vi "Main.vi"() -> ()   [LabVIEW 2017]
doc: "The program is for the real-time control of digital output pins on the Arduino Uno microcontroller.\n\nThe program is configured for the use of 6 DIO pins numbered 2-7. The pins can be be used to output AC and DC signals. The pins can also be swtiched on for a preset length of time."
uses:
  controls/UI Data.ctl
  <vilib>/MakerHub/LINX/Public/Peripherals/Digital/Digital Write 1 Chan.vi
  <vilib>/MakerHub/LINX/Public/Peripherals/Digital/Digital Write N Chans.vi
  <vilib>/MakerHub/LINX/Private/Local IO/LinxDigitalWrite.vi
  <vilib>/MakerHub/LINX/Public/Utilities/Check Channel.vi
  support/Message Queue/Enqueue Message (Single).vi
  <vilib>/MakerHub/LINX/Public/Utilities/Open Serial.vi
  <vilib>/MakerHub/LINX/Private/Utilties/Generate Error.vi
  <vilib>/Utility/error.llb/Error Cluster From Error Code.vi
  <vilib>/ErrorRing/Error Ring.xnode
  support/Message Queue/Message Queue.lvlib
  support/User Event - Stop/User Event - Stop.lvlib
  <vilib>/MakerHub/LINX/LMH-LINX.lvlib
panel:
  in  "Frequency (Hz)":dbl
  in  "DC/AC":bool
  in  "On-time (ms)":dbl
  in  "Start Button":bool
  in  "COM Port":refnum<visa-resource-name>="COM3"
  out "User Prompts":string="Initializing...."
  in  "Restart Button":bool
  in  "Exit":bool
  in  "Electrode Control":bool[][](array[boolean])=[[FALSE, FALSE, FALSE], [FALSE, FALSE, FALSE]]
  out "Error Out":errorcluster
  # "Digital Microfluidics HV Switching Control"
  # "Program Status"
  # "Timing Controls"
  # "DC"
  # "AC"
  # "Electrode Controls"
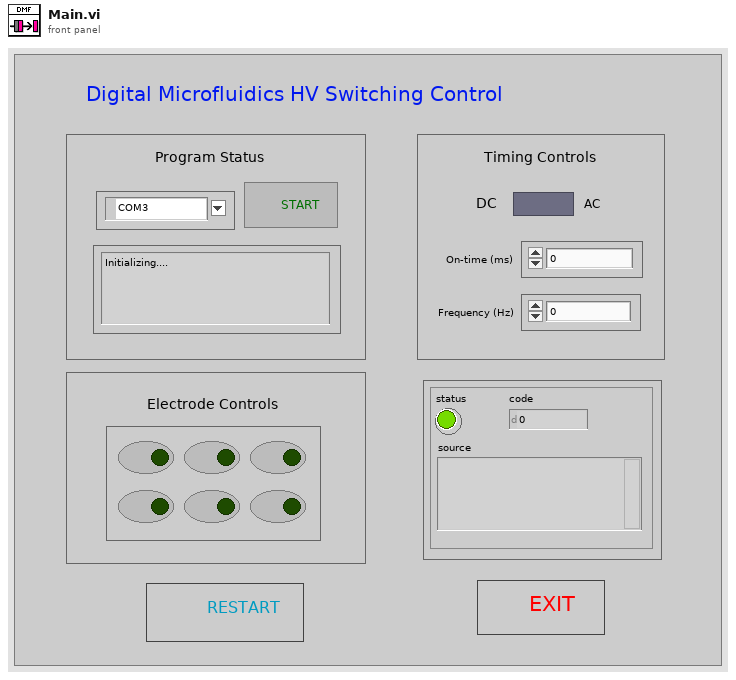
[diagram p1: front panel]
types:
  T1 = typedef "UI Data.ctl" = cluster{"VISA resource name":refnum<vi>, "Start Button":refnum<vi>, "DC/AC":refnum<vi>, "On-time (ms)":refnum<vi>, "Frequency (Hz)":refnum<vi>, "User Prompts":refnum<vi>, "Electrode Control":refnum<vi>, "Restart Button":refnum<vi>, "Exit":refnum<vi>}
  T2 = typedef "Message Queue.lvlib/All Message Queues.ctl" = cluster{"UI":refnum<queue>}
  T3 = typedef "LMH-LINX.lvlib/LINX Ref.ctl" = cluster{"IO":T4, "Interface":T5, "LINX Device Config":T6}
  T4 = typedef "LMH-LINX.lvlib/Platform.ctl" = enum16{"Remote", "Local"}
  T5 = typedef "LMH-LINX.lvlib/Interface.ctl" = enum16{"Serial", "TCP"}
  T6 = typedef "LMH-LINX.lvlib/Device.lvlib/LINX Device Config.ctl" = cluster{"Interface":T5, "COM Port":refnum<visa-resource-name>, "TCP Configuration":T7, "Device Family":u8, "Device ID":u8, "Device Name":string, "TCP Ref":refnum<k5>, "Channels":T8}
  T7 = typedef "LMH-LINX.lvlib/Device.lvlib/TCP Config.ctl" = cluster{"IP Address":string, "Port":u16}
  T8 = typedef "LMH-LINX.lvlib/Channels.ctl" = cluster{"DI":u8[], "DO":u8[], "AI":u8[], "AO":u8[], "PWM":u8[], "QE":u8[], "UART":u8[], "I2C 2":u8[], "SPI":u8[], "CAN":u8[], "Servo":u8[], "AI Ref (V)":dbl, "AI Resolution (Bits)":u8, "AO Ref (V)":dbl, "AO Resolution (Bits)":u8}
  T9 = cluster{i32, "index of element":i32, "Boolean":bool}
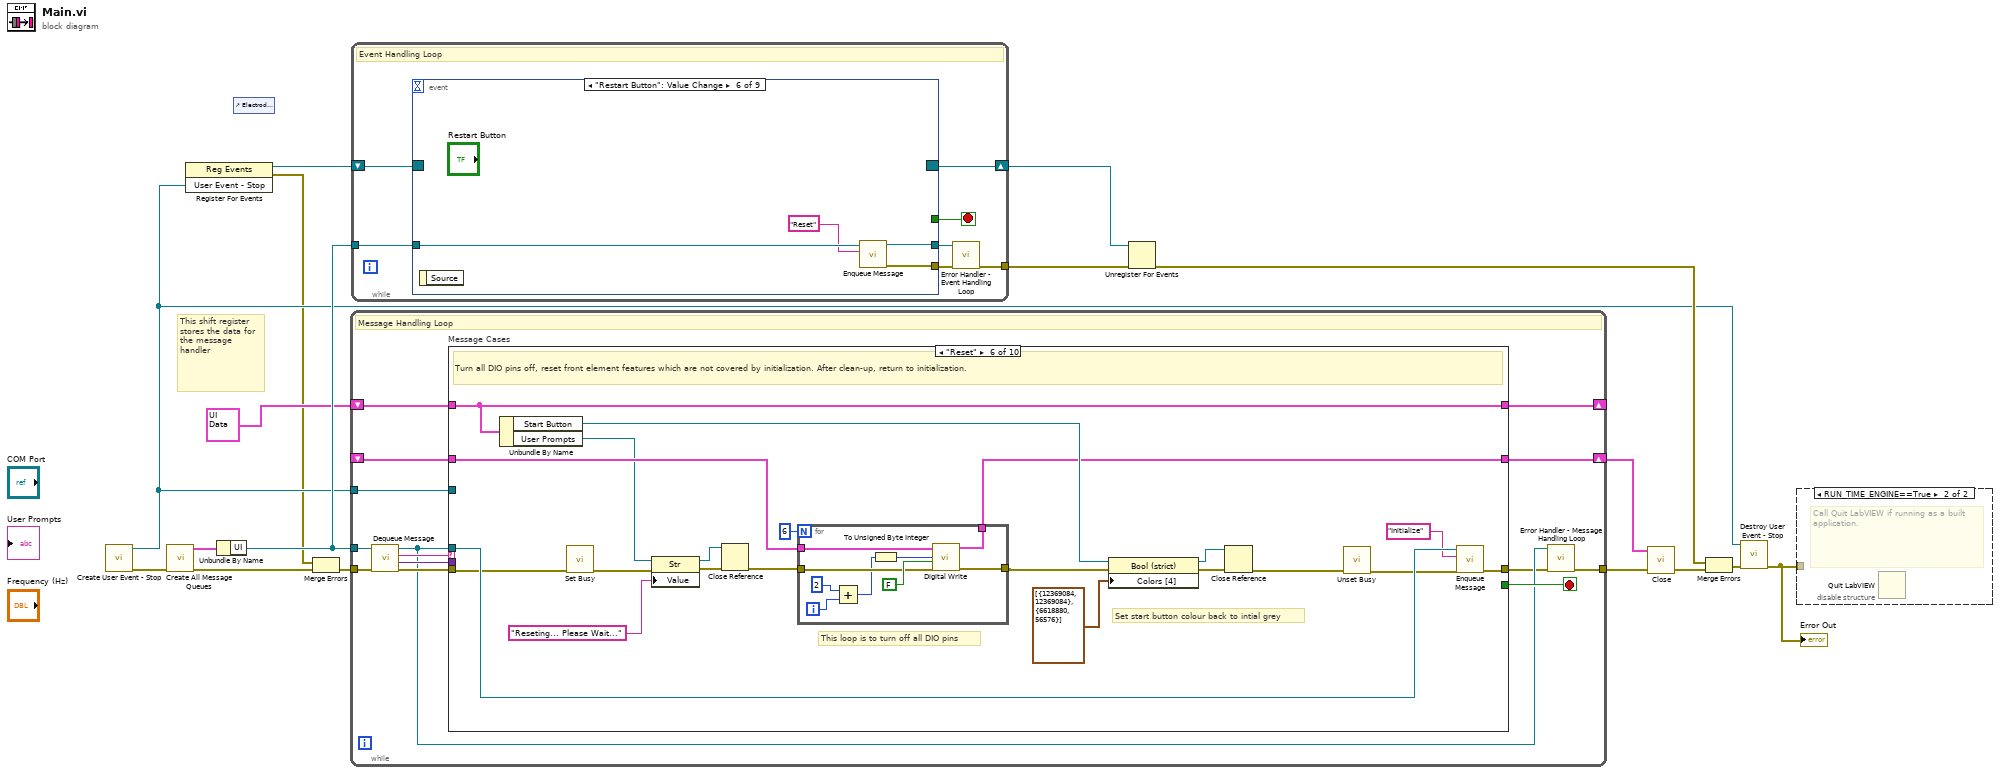
[diagram p0: block diagram]
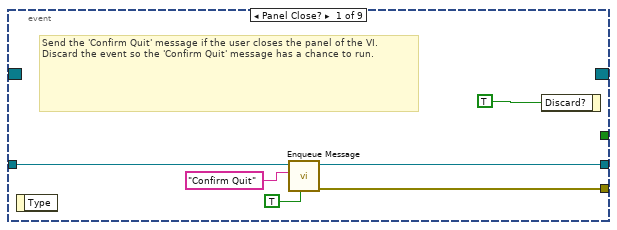
[diagram p3: hidden frame]
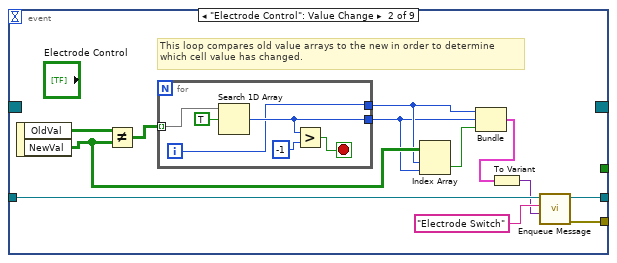
[diagram p4: hidden frame]
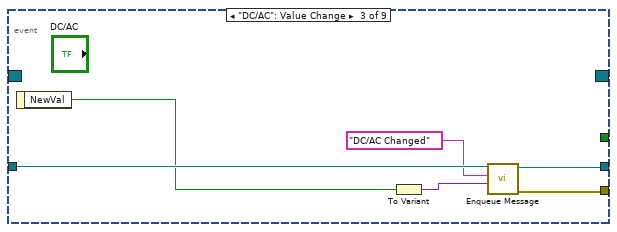
[diagram p5: hidden frame]
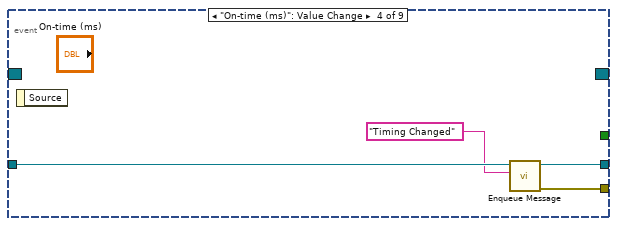
[diagram p6: hidden frame]
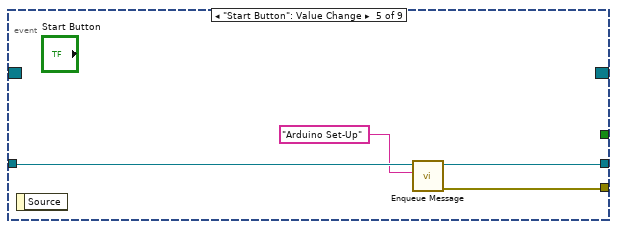
[diagram p7: hidden frame]
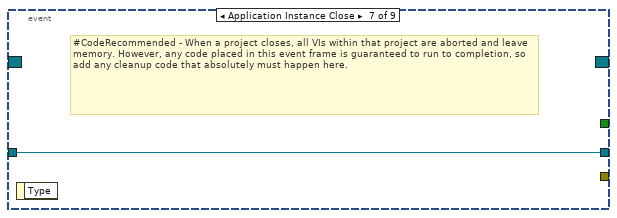
[diagram p8: hidden frame]
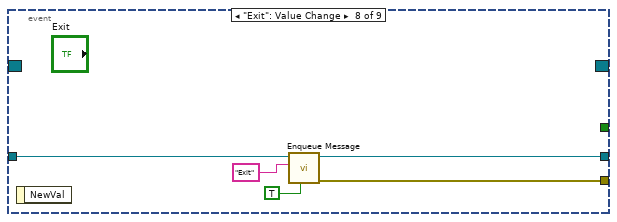
[diagram p9: hidden frame]
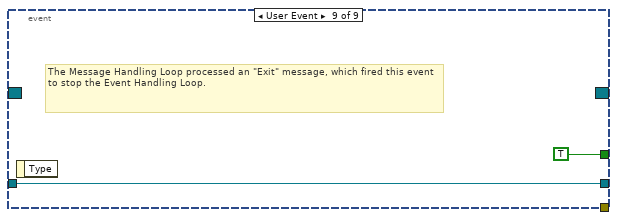
[diagram p10: hidden frame]
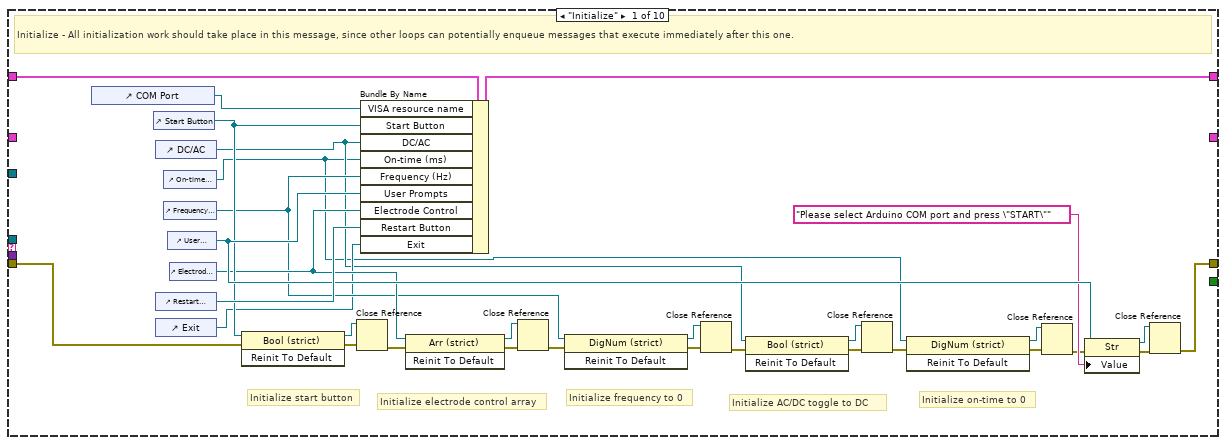
[diagram p11: hidden frame]
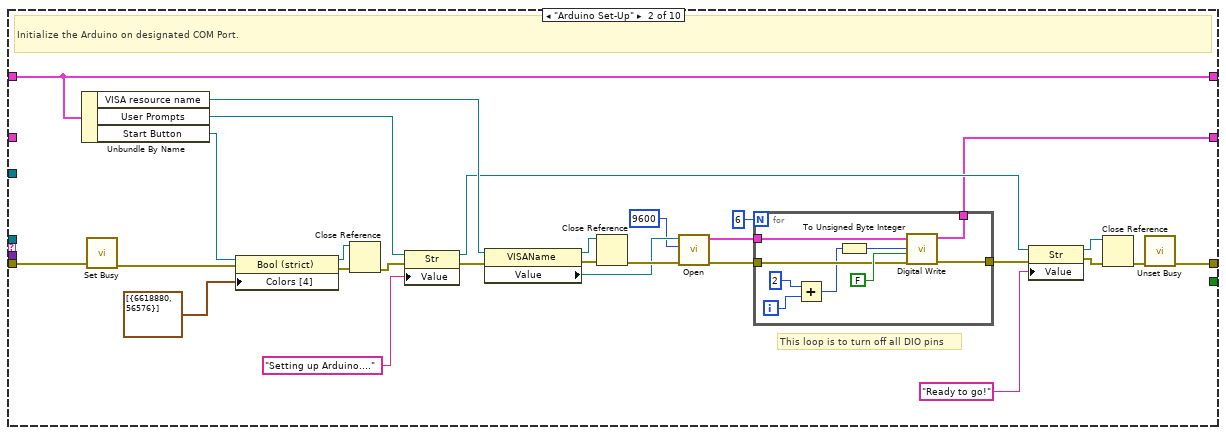
[diagram p12: hidden frame]
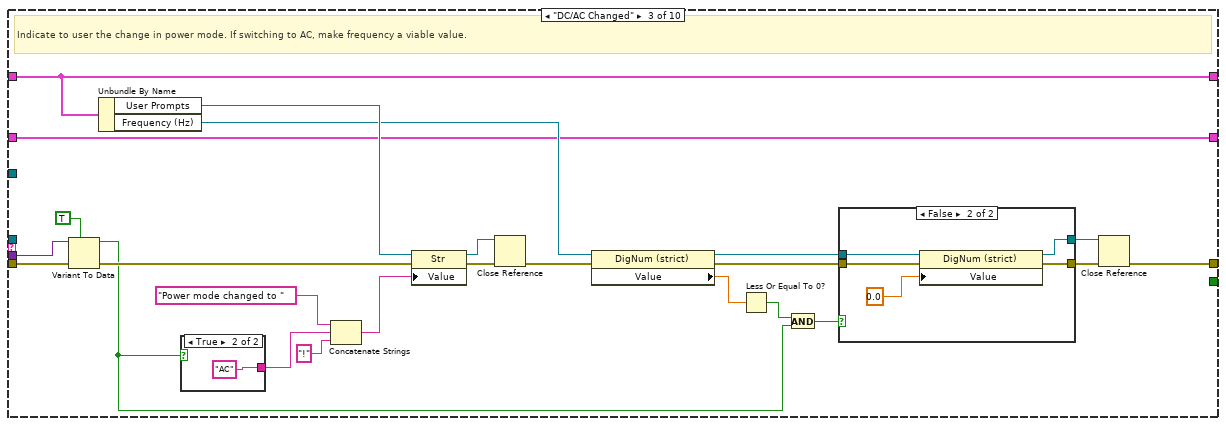
[diagram p13: hidden frame]
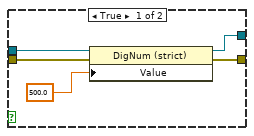
[diagram p14: hidden frame]
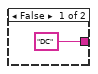
[diagram p15: hidden frame]
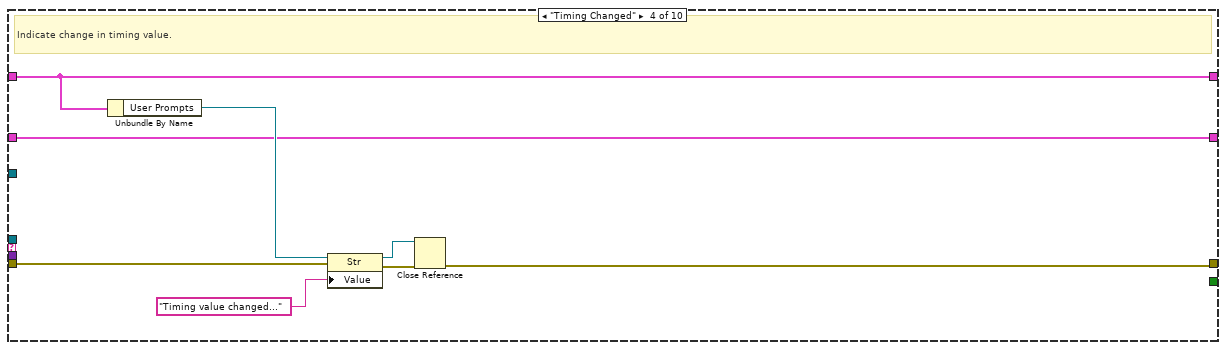
[diagram p16: hidden frame]
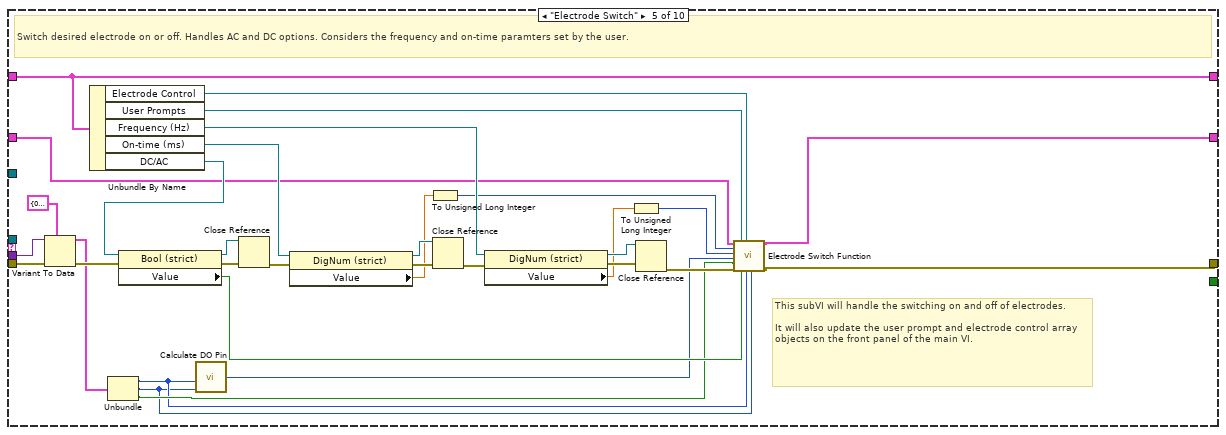
[diagram p17: hidden frame]
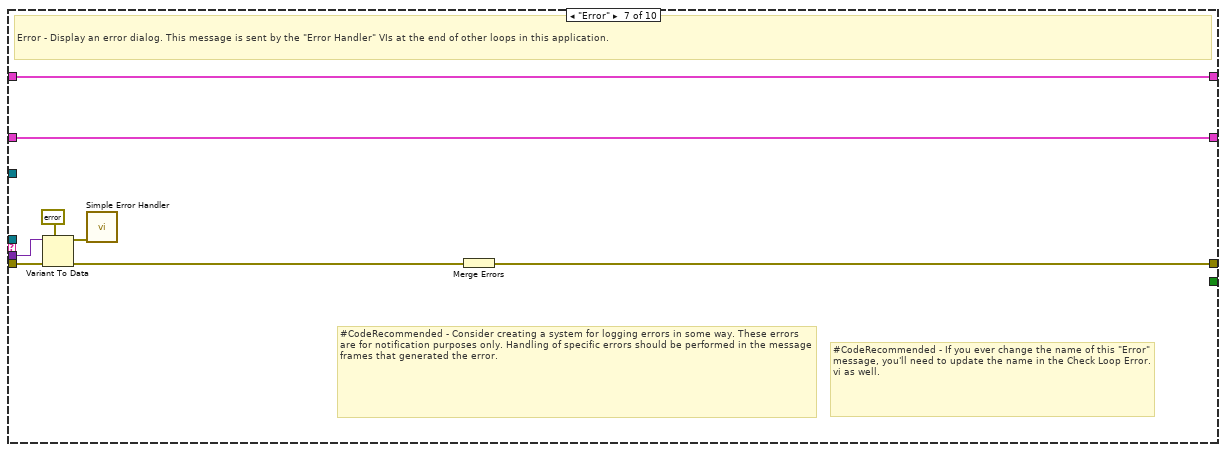
[diagram p18: hidden frame]
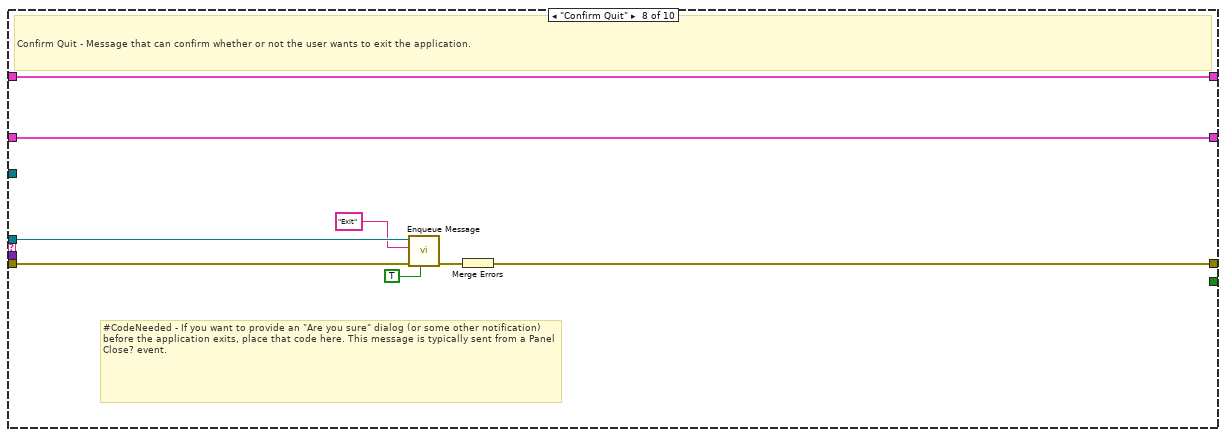
[diagram p19: hidden frame]
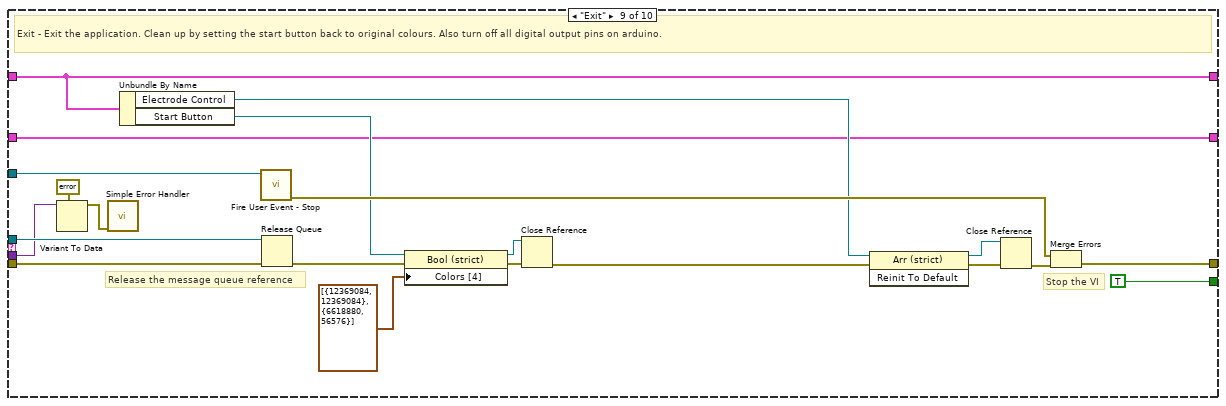
[diagram p20: hidden frame]
diagram:
  # "This shift register stores the data for the message handler"
  n1 = call "Create User Event - Stop.vi"() -> ("error out"=w14:errorcluster, "User Event - Stop"=w7:refnum<user-event>)  [unwired: 10 in]
  n2 = call "Create All Message Queues.vi"("error in (no error)"=w14) -> ("error out"=w17:errorcluster, "Message Queues out"=w16:T2)  [unwired: 9 in]
  n3 = register-events(w7) -> (reference out=w8:refnum<event-registration>, error out=w5:errorcluster)  [unwired: 2 in]
  n4 = Unbundle By Name(w16) -> ("UI"=w15:refnum<queue>)
  n5 = control-ref of="Electrode Control"() -> ()  [unwired: 1 out]
  n6 = Merge Errors(w5, w17) -> (w6:errorcluster)
  n7 = while {
    tunnel: w15 -> [w23]
    shift-right: [w30] -> _
    shift-left: T1 {"VISA resource name"=refnum, "Start Button"=refnum, "DC/AC"=refnum, "On-time (ms)"=refnum, "Frequency (Hz)"=refnum, "User Prompts"=refnum, "Electrode Control"=refnum, "Restart Button"=refnum, "Exit"=refnum} ("Data Cluster") -> [w31]
    tunnel: w7 -> [w28]
    tunnel: w6 -> [w27]
    tunnel: [w21] -> w3
    shift-right: [w19] -> w1
    shift-left: _ -> [w18]
    stop <- w29 stop-if-true
    # "Message Handling Loop"
    n8 = call "Dequeue Message.vi"("error in (no error)"=w27, "Message Queue"=w23) -> ("error out"=w26:errorcluster, "Message Data"=w24:variant, "Message"=w25:string, "dup Message Queue"=w22:refnum<queue>)  [unwired: 6 in]
    n9 = case "Message Cases" shown="\"Reset\"" w25 {
      selector: w25 -> [_ _ _ _ _ _ _ _ _ w244]
      tunnel: w22 -> [_ _ _ _ _ w187 _ w217 w242 _]
      tunnel: w26 -> [w53 w81 w122 w142 w175 w180 w213 w221 w237 _]
      tunnel: [w54 w79 w102 w138 w157 w188 w207 w219 w240 w245] -> w20
      tunnel: w31 -> [w62 w90 w123 w143 w172 w196 w212 w220 w233 w246]
      tunnel: [w61 w90 w123 w143 w172 w196 w212 w220 w233 w246] -> w30
      tunnel: [_ _ _ _ _ _ _ _ TRUE _] -> w29
      tunnel: w24 -> [_ _ w121 _ w174 _ w211 _ w234 _]
      tunnel: w28 -> [_ _ _ _ _ _ _ _ w239 _]
      tunnel: [_ w63 w100 w136 w156 w176 w206 w214 w223 w243] -> w19
      tunnel: w18 -> [_ _ w100 w136 w150 w194 w206 w214 w223 w243]
      frame "Initialize" {
        # "Initialize on-time to 0"
        # "Initialize AC/DC toggle to DC"
        # "Initialize frequency to 0"
        # "Initialize electrode control array"
        # "Initialize start button"
        # "Initialize - All initialization work should take place in this message, since other loops can potentially enqueue messages that execute immediately after this one."
        n10 = control-ref of="COM Port"() -> (w60:refnum<vi>)
        n11 = control-ref of="Start Button"() -> (w52:refnum<vi>)
        n12 = control-ref of="DC/AC"() -> (w39:refnum<vi>)
        n13 = control-ref of="Restart Button"() -> (w59:refnum<vi>)
        n14 = control-ref of="Exit"() -> (w41:refnum<vi>)
        n15 = control-ref of="On-time (ms)"() -> (w35:refnum<vi>)
        n16 = control-ref of="Frequency (Hz)"() -> (w44:refnum<vi>)
        n17 = control-ref of="User Prompts"() -> (w58:refnum<vi>)
        n18 = control-ref of="Electrode Control"() -> (w49:refnum<vi>)
        n19 = invoke class="Bool (strict)" method="Reinit To Default"(reference=w52, error in=w53) -> (reference out=w50:refnum<vi>, error out=w51:errorcluster)  [unwired: 1 in, 1 out]
        n20 = Close Reference(reference=w50, error in (no error)=w51) -> (error out=w48:errorcluster)
        n21 = Bundle By Name(cluster=w62, "VISA resource name"=w60, "Start Button"=w52, "DC/AC"=w39, "On-time (ms)"=w35, "Frequency (Hz)"=w44, "User Prompts"=w58, "Electrode Control"=w49, "Restart Button"=w59, "Exit"=w41) -> (w61:T1)
        n22 = invoke class="Arr (strict)" method="Reinit To Default"(reference=w49, error in=w48) -> (reference out=w46:refnum<vi>, error out=w47:errorcluster)  [unwired: 1 in, 1 out]
        n23 = Close Reference(reference=w46, error in (no error)=w47) -> (error out=w45:errorcluster)
        n24 = invoke class="DigNum (strict)" method="Reinit To Default"(reference=w44, error in=w45) -> (reference out=w42:refnum<vi>, error out=w43:errorcluster)  [unwired: 1 in, 1 out]
        n25 = Close Reference(reference=w42, error in (no error)=w43) -> (error out=w40:errorcluster)
        n26 = invoke class="Bool (strict)" method="Reinit To Default"(reference=w39, error in=w40) -> (reference out=w37:refnum<vi>, error out=w38:errorcluster)  [unwired: 1 in, 1 out]
        n27 = Close Reference(reference=w37, error in (no error)=w38) -> (error out=w36:errorcluster)
        n28 = invoke class="DigNum (strict)" method="Reinit To Default"(reference=w35, error in=w36) -> (reference out=w32:refnum<vi>, error out=w34:errorcluster)  [unwired: 1 in, 1 out]
        n29 = Close Reference(reference=w32, error in (no error)=w34) -> (error out=w33:errorcluster)
        n30 = property class="Str"(reference=w58, error in=w33, "Value"="Please select Arduino COM port and press \"START\"") -> (reference out=w56:refnum<vi>, error out=w57:errorcluster)
        n31 = Close Reference(reference=w56, error in (no error)=w57) -> (error out=w54:errorcluster)
      }
      frame "Arduino Set-Up" {
        # "This loop is to turn off all DIO pins"
        # "Initialize the Arduino on designated COM Port."
        n32 = Unbundle By Name(w90) -> ("VISA resource name"=w89:refnum<vi>, "User Prompts"=w83:refnum<vi>, "Start Button"=w72:refnum<vi>)
        n33 = call <vilib>:"Set Busy.vi"("error in (no error)"=w81) -> ("error out"=w73:errorcluster)  [unwired: 9 in, 1 out]
        n34 = property class="Bool (strict)"(reference=w72, error in=w73, "Colors [4]"=cluster{u32, u32}[] [{6618880, 56576}]) -> (reference out=w68:refnum<vi>, error out=w70:errorcluster)
        n35 = Close Reference(reference=w68, error in (no error)=w70) -> (error out=w69:errorcluster)
        n36 = property class="Str"(reference=w83, error in=w69, "Value"="Setting up Arduino....") -> (reference out=w77:refnum<vi>, error out=w78:errorcluster)
        n37 = property class="VISAName"(reference=w89, error in=w78) -> (reference out=w87:refnum<vi>, error out=w88:errorcluster, "Value"=w75:refnum<visa-resource-name>)
        n38 = Close Reference(reference=w87, error in (no error)=w88) -> (error out=w76:errorcluster)
        n39 = call-poly <vilib>:"Open.vi"("Error In"=w76, "Baud Rate Override"=u32 9600, "Serial Port"=w75) -> ("Error Out"=w66:errorcluster, "LINX Resource"=w64:T3)  [unwired: 6 in, 1 out]
        n40 = for {
          N: 6 -> [_]
          tunnel: [w99] -> w65
          tunnel: [w97] -> w63
          tunnel: w66 -> [w94]
          tunnel: w64 -> [w93]
          i -> [w96]
          n41 = Add(x=2, y=w96) -> (x+y=w91:i32)
          n42 = To Unsigned Byte Integer(number=w91) -> (unsigned 8bit integer=w92:u8)
          n43 = call-poly <vilib>:"Digital Write.vi"("Error In"=w94, "Output Value"=FALSE, "DO Channel"=w92, "LINX Resource"=w93) -> ("Error Out"=w99:errorcluster, "LINX Resource"=w97:T3)  [unwired: 6 in]
        }
        n44 = property class="Str"(reference=w77, error in=w65, "Value"="Ready to go!") -> (reference out=w85:refnum<vi>, error out=w86:errorcluster)
        n45 = Close Reference(reference=w85, error in (no error)=w86) -> (error out=w80:errorcluster)
        n46 = call <vilib>:"Unset Busy.vi"("error in (no error)"=w80) -> ("error out"=w79:errorcluster)  [unwired: 10 in]
      }
      frame "DC/AC Changed" {
        # "Indicate to user the change in power mode. If switching to AC, make frequency a viable value."
        n47 = Variant To Data(error in=w122, type=TRUE, Variant=w121) -> (data=w107:bool, error out=w117:errorcluster)
        n48 = Unbundle By Name(w123) -> ("User Prompts"=w114:refnum<vi>, "Frequency (Hz)"=w110:refnum<vi>)
        n49 = case shown="True" w107 {
          tunnel: ["DC" "AC"] -> w118
          frame False {
          }
          frame True {
          }
        }
        n50 = Concatenate Strings("Power mode changed to " ("string"), w118, "!") -> (w113:string)
        n51 = property class="Str"(reference=w114, error in=w117, "Value"=w113) -> (reference out=w115:refnum<vi>, error out=w116:errorcluster)
        n52 = Close Reference(reference=w115, error in (no error)=w116) -> (error out=w111:errorcluster)
        n53 = property class="DigNum (strict)"(reference=w110, error in=w111) -> (reference out=w104:refnum<vi>, error out=w105:errorcluster, "Value"=w109:dbl)
        n54 = Less Or Equal To 0?(x=w109) -> (x <= 0?=w108:bool)
        n55 = And(x=w108, y=w107) -> (x .and. y?=w106:bool)
        n56 = case shown="False" w106 {
          tunnel: w105 -> [w128 w133]
          tunnel: w104 -> [w127 w132]
          tunnel: [w125 w130] -> w103
          tunnel: [w124 w129] -> w101
          frame True {
            n57 = property class="DigNum (strict)"(reference=w127, error in=w128, "Value"=500.0) -> (reference out=w124:refnum<vi>, error out=w125:errorcluster)
          }
          frame False {
            n58 = property class="DigNum (strict)"(reference=w132, error in=w133, "Value"=0.0) -> (reference out=w129:refnum<vi>, error out=w130:errorcluster)
          }
        }
        n59 = Close Reference(reference=w101, error in (no error)=w103) -> (error out=w102:errorcluster)
      }
      frame "Timing Changed" {
        # "Indicate change in timing value."
        n60 = Unbundle By Name(w143) -> ("User Prompts"=w141:refnum<vi>)
        n61 = property class="Str"(reference=w141, error in=w142, "Value"="Timing value changed...") -> (reference out=w139:refnum<vi>, error out=w140:errorcluster)
        n62 = Close Reference(reference=w139, error in (no error)=w140) -> (error out=w138:errorcluster)
      }
      frame "Electrode Switch" {
        # "This subVI will handle the switching on and off of electrodes.\n\nIt will also update the user prompt and electrode control array objects on the front panel of the main VI."
        # "Switch desired electrode on or off. Handles AC and DC options. Considers the frequency and on-time paramters set by the user."
        n63 = Variant To Data(error in=w175, type=cluster{i32, i32, bool} {0, 0, FALSE}, Variant=w174) -> (data=w148:cluster{i32, i32, bool}, error out=w171:errorcluster)
        n64 = Unbundle By Name(w172) -> ("Electrode Control"=w146:refnum<vi>, "User Prompts"=w149:refnum<vi>, "Frequency (Hz)"=w160:refnum<vi>, "On-time (ms)"=w161:refnum<vi>, "DC/AC"=w162:refnum<vi>)
        n65 = Unbundle(w148) -> (w145:i32, w144:i32, w147:bool)
        n66 = property class="Bool (strict)"(reference=w162, error in=w171) -> (reference out=w169:refnum<vi>, error out=w170:errorcluster, "Value"=w155:bool)
        n67 = call "Calculate DO Pin.vi"("Row"=w145, "Col"=w144) -> ("MC Pin"=w153:u8)  [unwired: 3 in]
        n68 = Close Reference(reference=w169, error in (no error)=w170) -> (error out=w168:errorcluster)
        n69 = property class="DigNum (strict)"(reference=w161, error in=w168) -> (reference out=w166:refnum<vi>, error out=w167:errorcluster, "Value"=w165:dbl)
        n70 = To Unsigned Long Integer(number=w165) -> (unsigned 32bit integer=w151:u32)
        n71 = Close Reference(reference=w166, error in (no error)=w167) -> (error out=w159:errorcluster)
        n72 = property class="DigNum (strict)"(reference=w160, error in=w159) -> (reference out=w163:refnum<vi>, error out=w164:errorcluster, "Value"=w158:dbl)
        n73 = To Unsigned Long Integer(number=w158) -> (unsigned 32bit integer=w152:u32)
        n74 = Close Reference(reference=w163, error in (no error)=w164) -> (error out=w154:errorcluster)
        n75 = call "Electrode Switch Function.vi"("LINX Resource"=w150, "On-time (ms)"=w151, "Frequency"=w152, "Pin Number"=w153, "On or Off?"=w147, "Error In"=w154, "User Prompts Ref"=w149, "DC or AC?"=w155, "Electrode Control"=w146, "Row"=w145, "Column"=w144) -> ("LINX Resource Out"=w156:T3, "Error Out"=w157:errorcluster)  [unwired: 7 in]
      }
      frame "Reset" {
        # "Set start button colour back to intial grey"
        # "This loop is to turn off all DIO pins"
        # "Turn all DIO pins off, reset front element features which are not covered by initialization. After clean-up, return to initialization."
        n76 = Unbundle By Name(w196) -> ("Start Button"=w190:refnum<vi>, "User Prompts"=w183:refnum<vi>)
        n77 = call <vilib>:"Set Busy.vi"("error in (no error)"=w180) -> ("error out"=w179:errorcluster)  [unwired: 9 in, 1 out]
        n78 = property class="Str"(reference=w183, error in=w179, "Value"="Reseting... Please Wait...") -> (reference out=w182:refnum<vi>, error out=w185:errorcluster)
        n79 = Close Reference(reference=w182, error in (no error)=w185) -> (error out=w184:errorcluster)
        n80 = for {
          N: 6 -> [_]
          tunnel: [w205] -> w191
          tunnel: [w203] -> w176
          tunnel: w184 -> [w200]
          tunnel: w194 -> [w199]
          i -> [w202]
          n81 = Add(x=2, y=w202) -> (x+y=w197:i32)
          n82 = To Unsigned Byte Integer(number=w197) -> (unsigned 8bit integer=w198:u8)
          n83 = call-poly <vilib>:"Digital Write.vi"("Error In"=w200, "Output Value"=FALSE, "DO Channel"=w198, "LINX Resource"=w199) -> ("Error Out"=w205:errorcluster, "LINX Resource"=w203:T3)  [unwired: 6 in]
        }
        n84 = property class="Bool (strict)"(reference=w190, error in=w191, "Colors [4]"=cluster{u32, u32}[] [{12369084, 12369084}, {6618880, 56576}]) -> (reference out=w189:refnum<vi>, error out=w193:errorcluster)
        n85 = Close Reference(reference=w189, error in (no error)=w193) -> (error out=w177:errorcluster)
        n86 = call <vilib>:"Unset Busy.vi"("error in (no error)"=w177) -> ("error out"=w178:errorcluster)  [unwired: 10 in]
        n87 = call-poly "Enqueue Message.vi"("error in (no error)"=w178, "Message"="Initialize", "Message Queue"=w187) -> ("error out"=w188:errorcluster)  [unwired: 7 in, 1 out]
      }
      frame "Error" {
        # "#CodeRecommended - If you ever change the name of this \"Error\" message, you'll need to update the name in the Check Loop Error.vi as well."
        # "#CodeRecommended - Consider creating a system for logging errors in some way. These errors are for notification purposes only. Handling of specific errors should be performed in the message frames that generated the error."
        # "Error - Display an error dialog. This message is sent by the \"Error Handler\" VIs at the end of other loops in this application."
        n88 = Variant To Data(error in=w213, type=errorcluster {"status"=FALSE, "code"=0, "source"=""} ("error constant"), Variant=w211) -> (data=w209:errorcluster, error out=w208:errorcluster)
        n89 = call <vilib>:"Simple Error Handler.vi"("error in (no error)"=w209) -> ()  [unwired: 4 in, 5 out]
        n90 = Merge Errors(w208) -> (w207:errorcluster)
      }
      frame "Confirm Quit" {
        # "#CodeNeeded - If you want to provide an \"Are you sure\" dialog (or some other notification) before the application exits, place that code here. This message is typically sent from a Panel Close? event."
        # "Confirm Quit - Message that can confirm whether or not the user wants to exit the application."
        n91 = call-poly "Enqueue Message.vi"("Priority Message? (F)"=TRUE, "error in (no error)"=w221, "Message"="Exit", "Message Queue"=w217) -> ("error out"=w218:errorcluster)  [unwired: 6 in, 1 out]
        n92 = Merge Errors(w218) -> (w219:errorcluster)
      }
      frame "Exit" {
        # "Stop the VI"
        # "Release the message queue reference"
        # "Exit - Exit the application. Clean up by setting the start button back to original colours. Also turn off all digital output pins on arduino."
        n93 = Variant To Data(type=errorcluster {"status"=FALSE, "code"=0, "source"=""} ("error constant"), Variant=w234) -> (data=w235:errorcluster)  [unwired: 1 in, 1 out]
        n94 = call <vilib>:"Simple Error Handler.vi"("error in (no error)"=w235) -> ()  [unwired: 4 in, 5 out]
        n95 = Unbundle By Name(w233) -> ("Electrode Control"=w225:refnum<vi>, "Start Button"=w228:refnum<vi>)
        n96 = call "Fire User Event - Stop.vi"("User Event - Stop"=w239) -> ("error out"=w238:errorcluster)  [unwired: 10 in]
        n97 = Release Queue(queue=w242, error in (no error)=w237) -> (error out=w232:errorcluster)  [unwired: 1 in, 2 out]
        n98 = property class="Bool (strict)"(reference=w228, error in=w232, "Colors [4]"=cluster{u32, u32}[] [{12369084, 12369084}, {6618880, 56576}]) -> (reference out=w230:refnum<vi>, error out=w231:errorcluster)
        n99 = Close Reference(reference=w230, error in (no error)=w231) -> (error out=w222:errorcluster)
        n100 = invoke class="Arr (strict)" method="Reinit To Default"(reference=w225, error in=w222) -> (reference out=w224:refnum<vi>, error out=w227:errorcluster)  [unwired: 1 in, 1 out]
        n101 = Close Reference(reference=w224, error in (no error)=w227) -> (error out=w226:errorcluster)
        n102 = Merge Errors(w238, w226) -> (w240:errorcluster)
      }
      frame Default {
        # "'Default' case only runs if there is a message that isn't defined in any of the other cases.  Output a programming error."
        n103 = xnode "Error Ring"("parameter 0"=w244) -> ("error out"=w245:errorcluster)
      }
    }
    n104 = call "Error Handler - Message Handling Loop.vi"("error in (no error)"=w20, "Message Queue"=w22) -> ("dup error in"=w21:errorcluster)  [unwired: 8 in, 1 out]
  }
  n105 = while {
    tunnel: w15 -> [w260]
    shift-right: [w258] -> w11
    shift-left: w8 -> [w259]
    tunnel: [w254] -> w9
    stop <- w256 stop-if-true
    # "Event Handling Loop"
    n106 = event shown="[5] \"Restart Button\": Value Change" {
      selector: w259 -> [_ _ _ _ _ _ _ _ _]
      dyn-events: [_ _ _ _ _ _ _ _ _] -> w258
      timeout: _ -> [_ _ _ _ _ _ _ _ _]
      tunnel: [_ _ _ _ _ _ _ _ TRUE ("Discard?")] -> w256
      tunnel: w260 -> [w265 w278 w289 w292 w297 w302 w303 w308 w310]
      tunnel: [w264 w276 w290 w293 w296 w300 _ w307 _] -> w257
      tunnel: [w263 w277 w288 w294 w298 w301 w303 w306 w310] -> w255
      event Panel Close? {
        # "Send the 'Confirm Quit' message if the user closes the panel of the VI. Discard the event so the 'Confirm Quit' message has a chance to run."
        n107 = event-data() -> ()  [unwired: 1 in, 1 out]
        n108 = call-poly "Enqueue Message.vi"("Priority Message? (F)"=TRUE, "Message"="Confirm Quit", "Message Queue"=w265) -> ("error out"=w264:errorcluster, "dup Message Queue"=w263:refnum<queue>)  [unwired: 7 in]
        n109 = event-data("Discard?"=TRUE) -> ()  [unwired: 1 in, 1 out]
      }
      event "Electrode Control": Value Change {
        # "This loop compares old value arrays to the new in order to determine\nwhich cell value has changed."
        n110 = event-data() -> ("OldVal"=w275:bool[][], "NewVal"=w272:bool[][])  [unwired: 1 in]
        n111 = Not Equal?(x=w275, y=w272) -> (x != y?=w274:bool[][])
        n112 = for {
          tunnel: w274 -> [w284] mode=indexing
          tunnel: [w282] -> w267
          tunnel: [w279] -> w268
          i -> [w279]
          stop <- w280 stop-if-true
          n113 = Search 1D Array(1D array=w284, element=TRUE) -> (index of element=w282:i32)  [unwired: 1 in]
          n114 = Greater?(x=w282, y=-1) -> (0:w280:bool)
        }
        n115 = Index Array(array=w272, index (row)=w268, index (col)=w267) -> (element=w271:bool)
        n116 = Bundle(w268, "index of element"=w267, "Boolean"=w271) -> (w270:T9)  [unwired: 1 in]
        n117 = To Variant(anything=w270) -> (Variant=w269:variant)
        n118 = call-poly "Enqueue Message.vi"("Message Data"=w269, "Message"="Electrode Switch", "Message Queue"=w278) -> ("error out"=w276:errorcluster, "dup Message Queue"=w277:refnum<queue>)  [unwired: 7 in]
      }
      event "DC/AC": Value Change {
        n119 = event-data() -> ("NewVal"=w287:bool)  [unwired: 1 in]
        n120 = To Variant(anything=w287) -> (Variant=w286:variant)
        n121 = call-poly "Enqueue Message.vi"("Message Data"=w286, "Message"="DC/AC Changed", "Message Queue"=w289) -> ("error out"=w290:errorcluster, "dup Message Queue"=w288:refnum<queue>)  [unwired: 7 in]
      }
      event "On-time (ms)": Value Change {
        n122 = event-data() -> ()  [unwired: 1 in, 1 out]
        n123 = call-poly "Enqueue Message.vi"("Message"="Timing Changed", "Message Queue"=w292) -> ("error out"=w293:errorcluster, "dup Message Queue"=w294:refnum<queue>)  [unwired: 8 in]
      }
      event "Start Button": Value Change {
        n124 = event-data() -> ()  [unwired: 1 in, 1 out]
        n125 = call-poly "Enqueue Message.vi"("Message"="Arduino Set-Up", "Message Queue"=w297) -> ("error out"=w296:errorcluster, "dup Message Queue"=w298:refnum<queue>)  [unwired: 8 in]
      }
      event "Restart Button": Value Change {
        n126 = event-data() -> ()  [unwired: 1 in, 1 out]
        n127 = call-poly "Enqueue Message.vi"("Message"="Reset", "Message Queue"=w302) -> ("error out"=w300:errorcluster, "dup Message Queue"=w301:refnum<queue>)  [unwired: 8 in]
      }
      event Application Instance Close {
        # "#CodeRecommended - When a project closes, all VIs within that project are aborted and leave memory. However, any code placed in this event frame is guaranteed to run to completion, so add any cleanup code that absolutely must happen here."
        n128 = event-data() -> ()  [unwired: 1 in, 1 out]
      }
      event "Exit": Value Change {
        n129 = event-data() -> ()  [unwired: 1 in, 1 out]
        n130 = call-poly "Enqueue Message.vi"("Priority Message? (F)"=TRUE, "Message"="Exit", "Message Queue"=w308) -> ("error out"=w307:errorcluster, "dup Message Queue"=w306:refnum<queue>)  [unwired: 7 in]
      }
      event User Event {
        # "The Message Handling Loop processed an \"Exit\" message, which fired this event to stop the Event Handling Loop."
        n131 = event-data() -> ()  [unwired: 1 in, 1 out]
      }
    }
    n132 = call "Error Handler - Event Handling Loop.vi"("error in (no error)"=w257, "Message Queue"=w255) -> ("dup error in"=w254:errorcluster)  [unwired: 8 in, 1 out]
  }
  n133 = Unregister For Events(event registration refnum=w11, error in=w9) -> (error out=w12:errorcluster)
  n134 = call <vilib>:"Close.vi"("Error In"=w3, "LINX Resource"=w1) -> ("Error Out"=w2:errorcluster)  [unwired: 9 in]
  n135 = Merge Errors(w12, w2) -> (w13:errorcluster)
  n136 = call "Destroy User Event - Stop.vi"("error in (no error)"=w13, "User Event - Stop"=w7) -> ("error out"=w4:errorcluster)  [unwired: 9 in]
  "Error Out" <- w4
  n137 = disable-structure shown="RUN_TIME_ENGINE==True" {
    disable-tunnel: w4 -> [_ _]
    frame condition #0 (active) {
    }
    frame condition #1 {
      # "Call Quit LabVIEW if running as a built application."
      n138 = Quit LabVIEW() -> ()  [unwired: 1 in]
    }
  }
